vi "PosBolaFora.vi"(9 "Field Size in":T1, 10 "Position da bola":dbl[](array[numeric]), 11 "Position do robot":dbl[](array[numeric])) -> (3 "Target":dbl[](array[numeric]))   [LabVIEW 2016]
uses:
  Core/Field Size.ctl
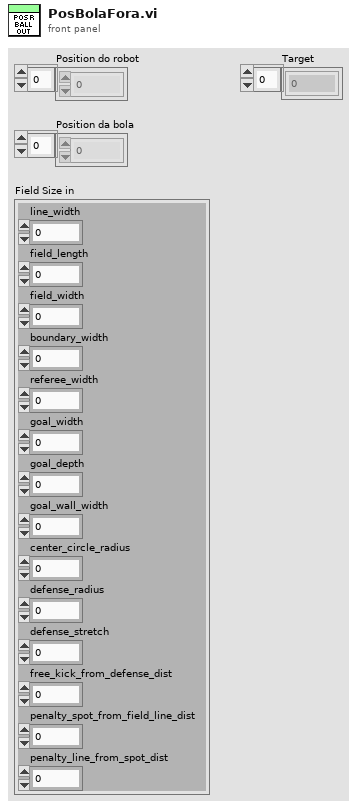
[diagram p1: front panel]
types:
  T1 = typedef "Field Size.ctl" = cluster{"line_width":u32, "field_length":u32, "field_width":u32, "boundary_width":u32, "referee_width":u32, "goal_width":u32, "goal_depth":u32, "goal_wall_width":u32, "center_circle_radius":u32, "defense_radius":u32, "defense_stretch":u32, "free_kick_from_defense_dist":u32, "penalty_spot_from_field_line_dist":u32, "penalty_line_from_spot_dist":u32}
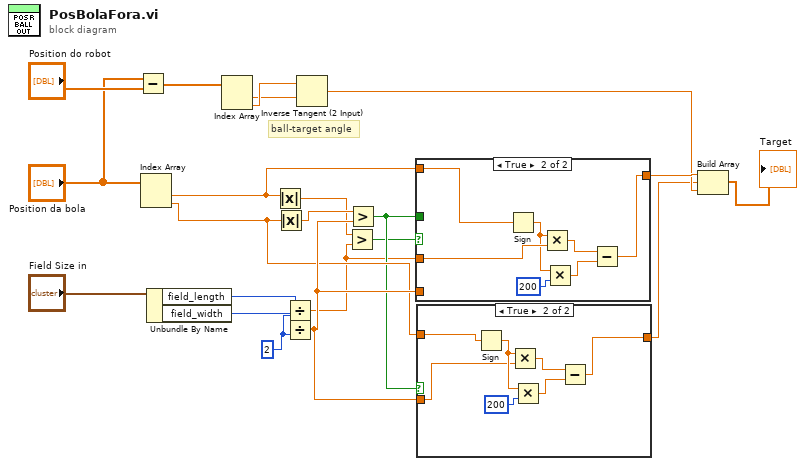
[diagram p0: block diagram]
diagram:
  w4 = u32 2 ("y")
  # "ball-target angle"
  n1 = Subtract(x="Position da bola", y="Position do robot") -> (x-y=w11:dbl[])
  n2 = Index Array(array="Position da bola") -> (element #1=w8:dbl, element #2=w18:dbl)  [unwired: 2 in]
  n3 = Unbundle By Name("Field Size in") -> ("field_length"=w2:u32, "field_width"=w3:u32)
  n4 = Index Array(array=w11) -> (element #1=w9:dbl, element #2=w10:dbl)  [unwired: 2 in]
  n5 = Absolute Value(x=w8) -> (abs(x)=w5:dbl)
  n6 = Absolute Value(x=w18) -> (abs(x)=w7:dbl)
  n7 = Divide(x=w2, y=w4) -> (x/y=w14:dbl)
  n8 = Divide(x=w3, y=w4) -> (x/y=w19:dbl)
  n9 = Inverse Tangent (2 Input)(1:w9, 2:w10) -> (0:w12:dbl)
  n10 = Greater?(x=w5, y=w14) -> (0:w6:bool)
  n11 = Greater?(x=w7, y=w19) -> (0:w17:bool)
  n12 = case shown="True" w6 {
    tunnel: w17 -> [_ _]
    tunnel: w8 -> [w22 w29]
    tunnel: [w22 w27] -> w13
    tunnel: w14 -> [_ w28]
    tunnel: w19 -> [_ _]
    frame False {
    }
    frame True {
      n13 = Sign(1:w29) -> (0:w24:dbl)
      n14 = Multiply(x=w24, y=w28) -> (x*y=w26:dbl)
      n15 = Multiply(x=w24, y=200) -> (x*y=w23:dbl)
      n16 = Subtract(x=w26, y=w23) -> (x-y=w27:dbl)
    }
  }
  n17 = case shown="True" w17 {
    tunnel: w18 -> [w30 w33]
    tunnel: w19 -> [_ w31]
    tunnel: [w30 w32] -> w1
    frame False {
    }
    frame True {
      n18 = Sign(1:w33) -> (0:w35:dbl)
      n19 = Multiply(x=w35, y=w31) -> (x*y=w37:dbl)
      n20 = Multiply(x=w35, y=200) -> (x*y=w34:dbl)
      n21 = Subtract(x=w37, y=w34) -> (x-y=w32:dbl)
    }
  }
  n22 = Build Array(w13, w1, w12) -> (→"Target":dbl[])
